vi "Measurement UI.vi"() -> ()   [LabVIEW 2021, in "ImageRendering.lvlib"]
uses:
  ImageRendering.lvlib
  <vilib>/vision/Image Controls.llb/IMAQ Image.ctl
  nivissvc.dll
  nivision.dll
panel:
  out "Time taken to receive image (seconds)":dbl
  out "Image Acq time":string
  out "Image Pixels (U32)":u32[](array[numeric])
  in  "Image Pixels (U64) 2":T1[][](array[typedef])
  in  "Image Converison Type":string(combo)="ImagePixelArray"
  out "Image Data Received":string
  out "value":u32[][](array[numeric])
  out "Image":T2(plugin-control)
  in  "Border Size":i32=3
  in  "Image Name":string="copy"
  in  "Image Type":u32(ring)=4 items=["Grayscale (U8)", "Grayscale (I16)", "Grayscale (SGL)", "Complex (CSG)", "RGB (U32)", "HSL (U32)", "RGB (U64)", "Grayscale (U16)"]
  out "File Size":dbl
  out "error out":errorcluster
  out "date/time string":string
  in  "Image Path":path
  out "Image Data":string
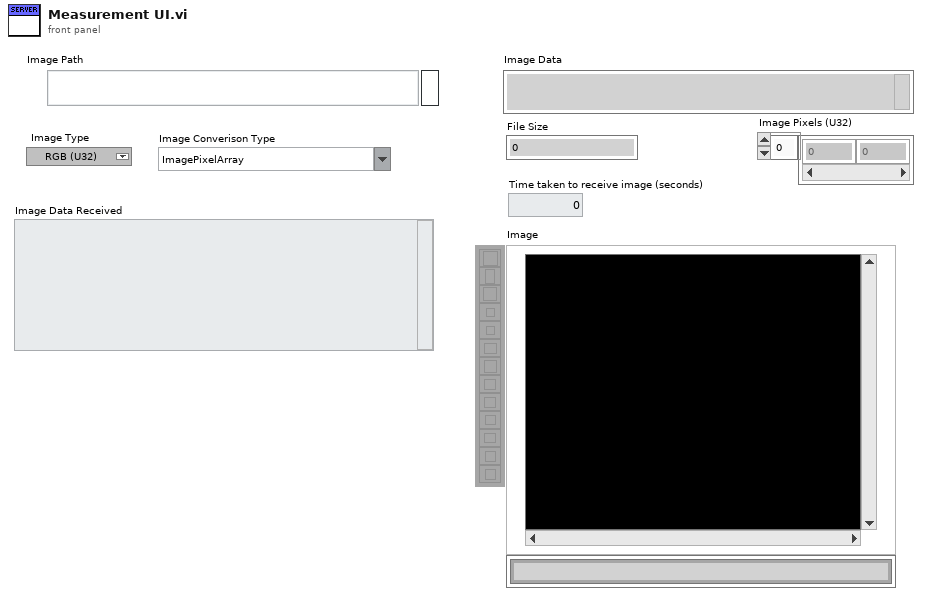
[diagram p1: front panel]
types:
  T1 = typedef "Color (U64)" = cluster{"Plane 3 (Blue)":u16, "Plane 2 (Green)":u16, "Plane 1 (Red)":u16, "Plane 4 (alpha)":u16}
  T2 = typedef "IMAQ Image.ctl" = refnum<image>
  T3 = enum16{"open", "replace", "create", "open or create", "replace or create", "replace or create with confirmation"}
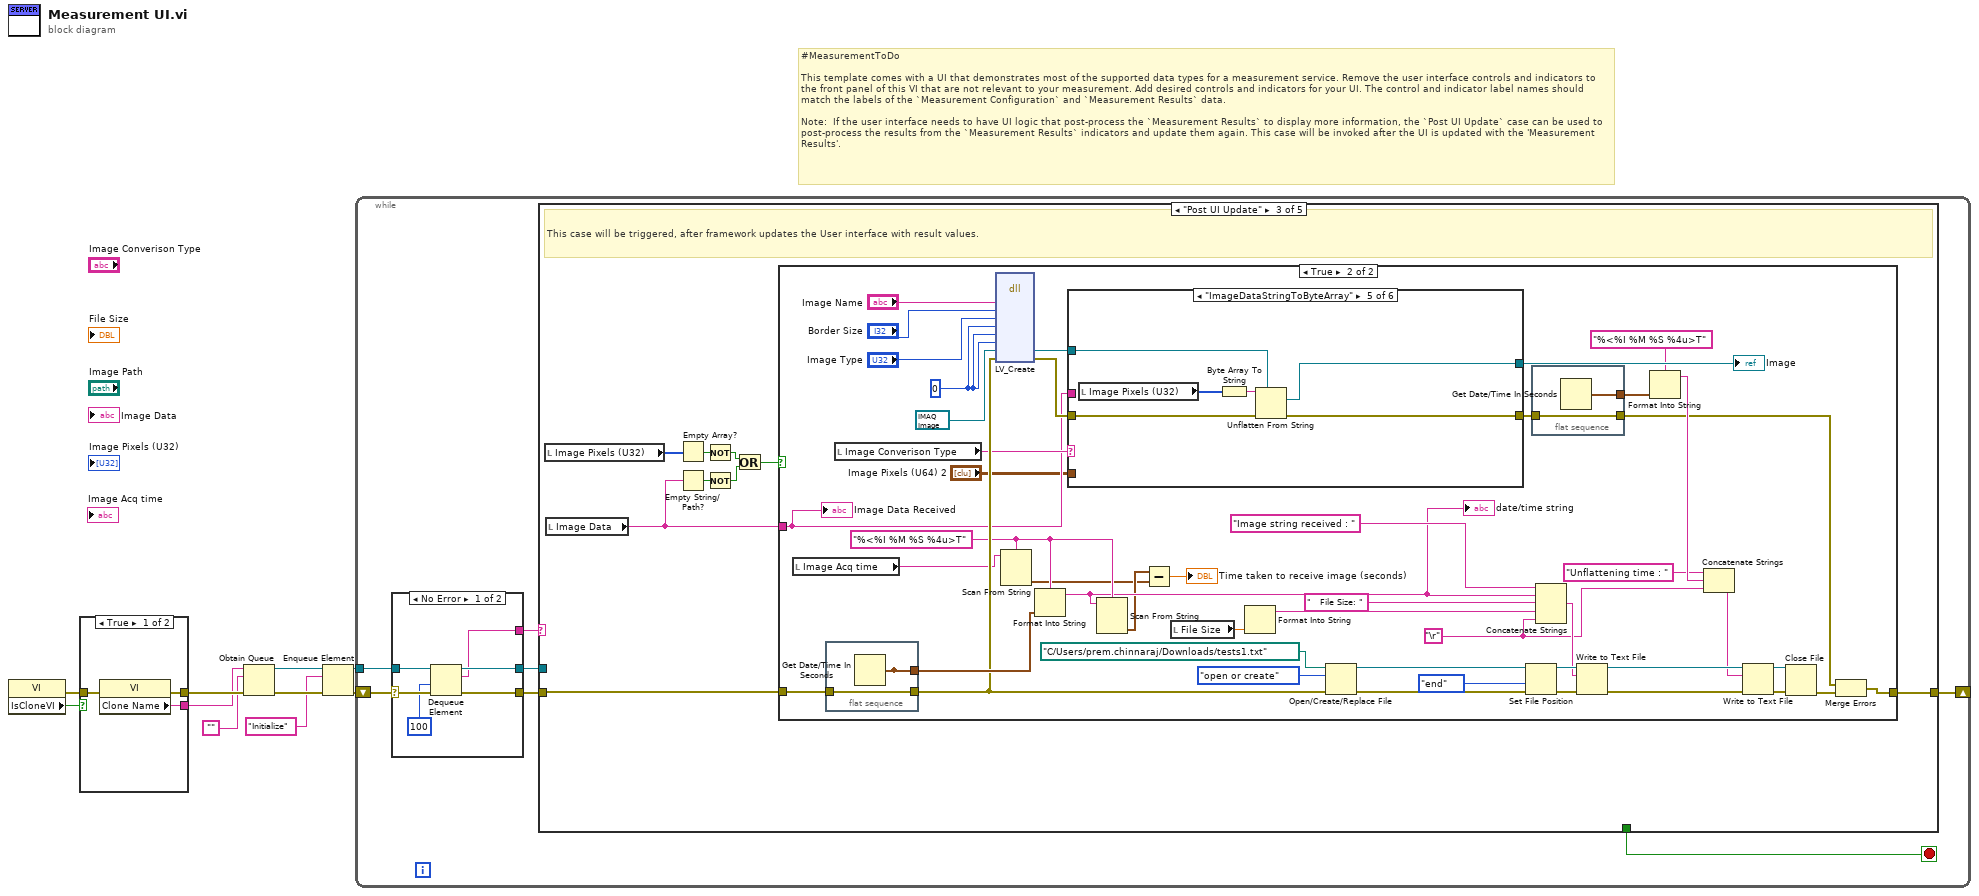
[diagram p0: block diagram]
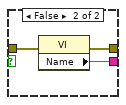
[diagram p2: hidden frame]
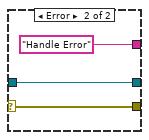
[diagram p3: hidden frame]
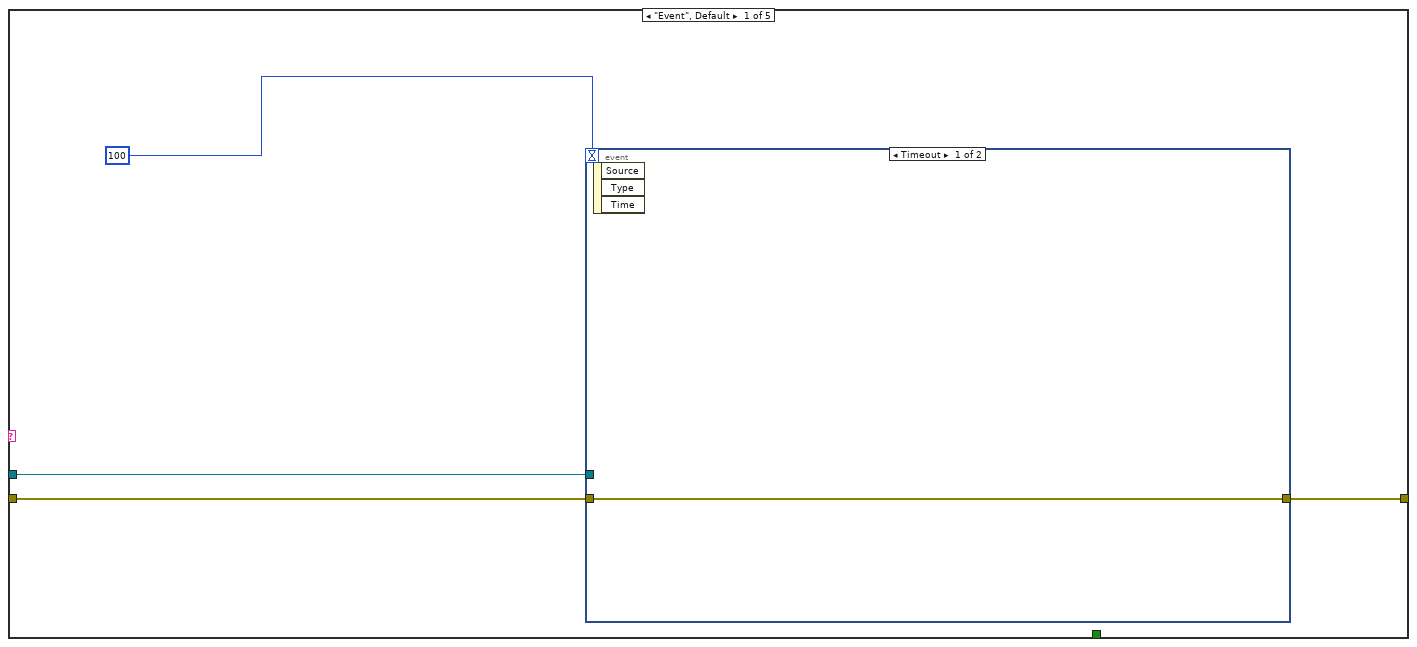
[diagram p4: hidden frame]
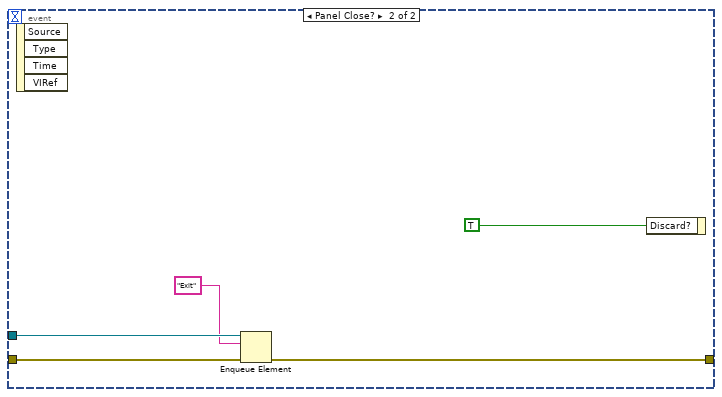
[diagram p5: hidden frame]
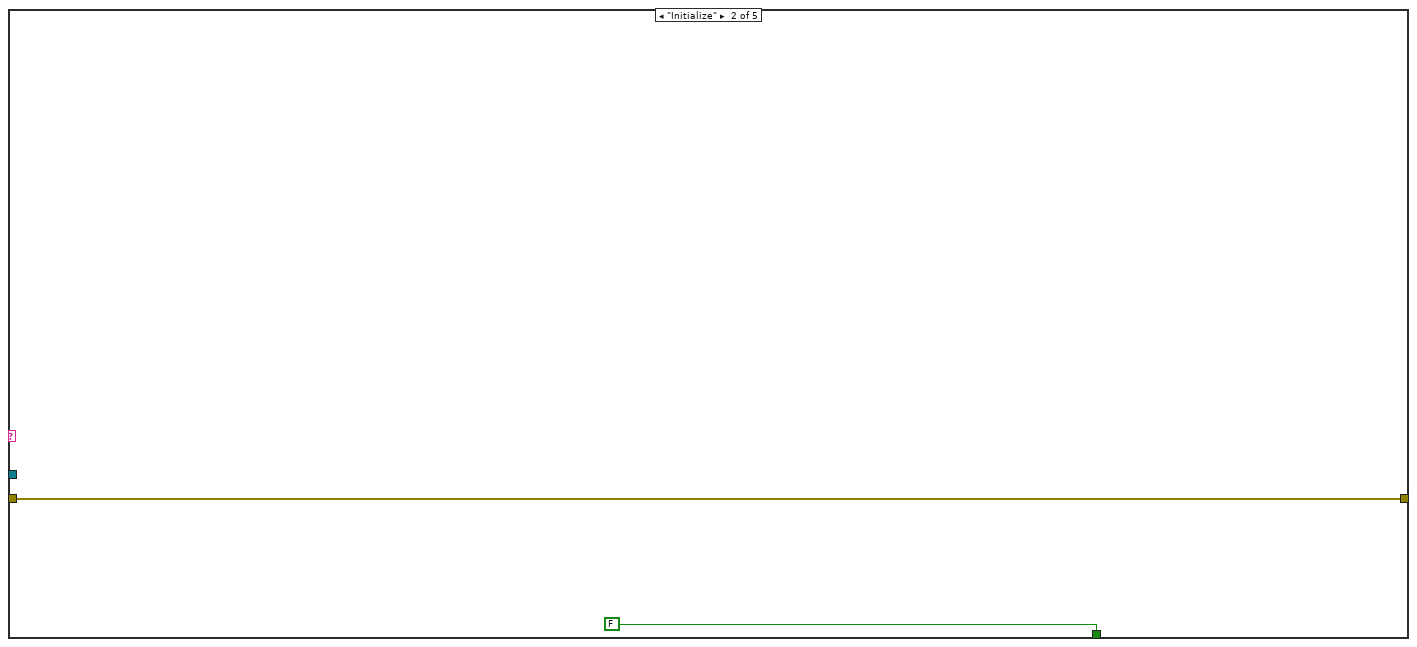
[diagram p6: hidden frame]
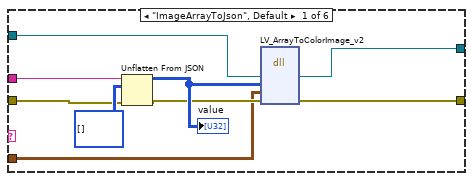
[diagram p8: hidden frame]
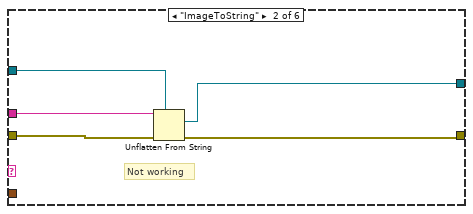
[diagram p9: hidden frame]
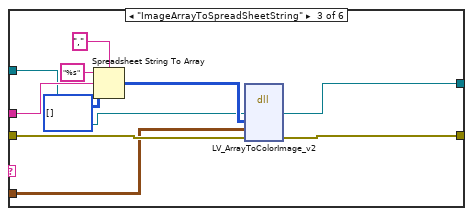
[diagram p10: hidden frame]
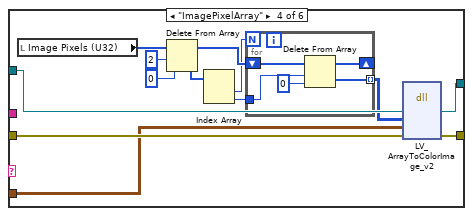
[diagram p11: hidden frame]
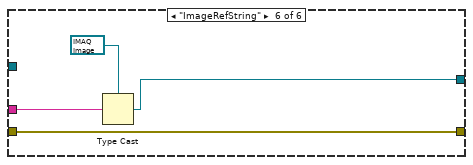
[diagram p12: hidden frame]
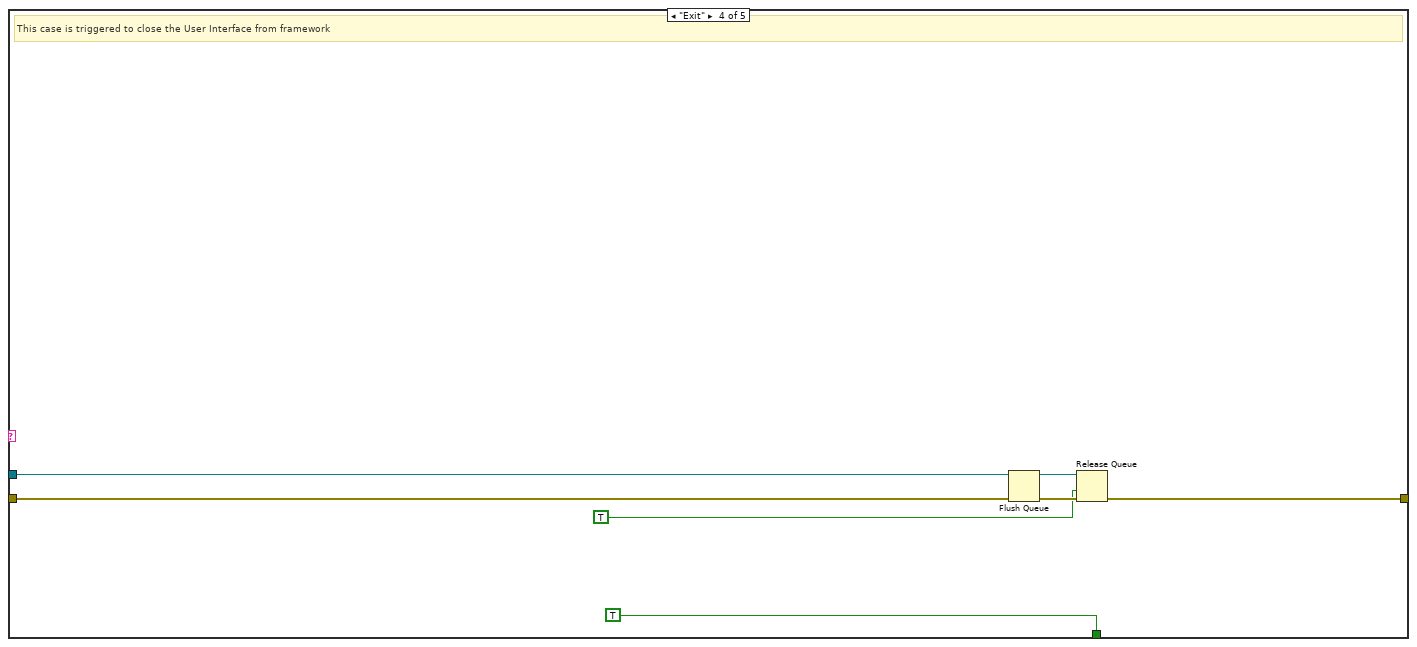
[diagram p13: hidden frame]
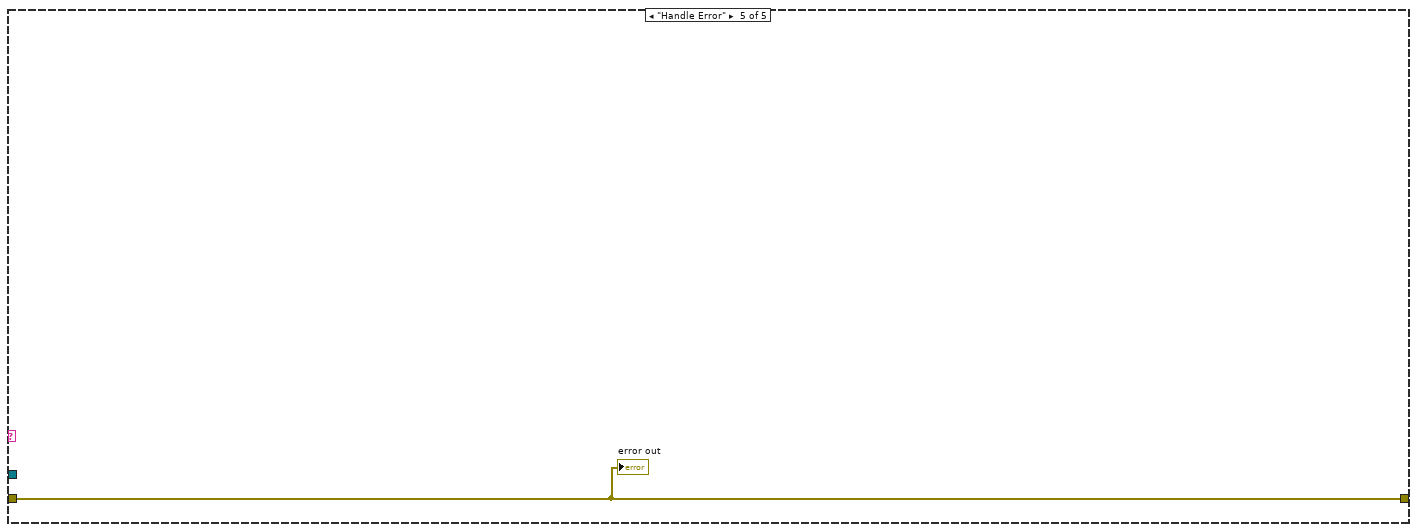
[diagram p14: hidden frame]
diagram:
  # "#MeasurementToDo  \n\nThis template comes with a UI that demonstrates most of the supported data types for a measurement service. Remove the user interface controls and indicators to the front panel of this VI that are not relevant to your measurement. Add desired controls and indicators for your UI. The control and indicator label names should match the labels of the `Measurement Configuration` and `Measurement Results` data.\n\nNote:  If the user interface needs to have UI logic that post-process the `Measurement Results` to display more information, the `Post UI Update` case can be used to post-process the results from the `Measurement Results` indicators and update them again. This case will be invoked after the UI is updated with the 'Measurement Results'."
  n1 = property class="VI"() -> (error out=w1:errorcluster, "IsCloneVI"=w2:bool)  [unwired: 2 in, 1 out]
  n2 = case shown="True" w2 {
    tunnel: [w13 w16] -> w10
    tunnel: [w12 w15] -> w9
    tunnel: w1 -> [w11 w14]
    frame True {
      n3 = property class="VI"(error in=w11) -> (error out=w13:errorcluster, "Clone Name"=w12:string)  [unwired: 1 in, 1 out]
    }
    frame False {
      n4 = property class="VI"(error in=w14) -> (error out=w16:errorcluster, "Name"=w15:string)  [unwired: 1 in, 1 out]
    }
  }
  n5 = Obtain Queue(name (unnamed)=w9, element data type="", error in (no error)=w10) -> (queue out=w6:refnum<queue>, error out=w8:errorcluster)  [unwired: 2 in, 1 out]
  n6 = Enqueue Element(queue=w6, element="Initialize", error in (no error)=w8) -> (queue out=w5:refnum<queue>, error out=w7:errorcluster)  [unwired: 1 in, 1 out]
  n7 = while {
    shift-right: [w19] -> _
    shift-left: w7 -> [w23]
    tunnel: w5 -> [w22]
    stop <- w18 stop-if-true
    n8 = case shown="No Error" w23 {
      selector: w23 -> [w29 w32]
      tunnel: [w28 w32] -> w17
      tunnel: w22 -> [w27 w31]
      tunnel: [w26 w31] -> w21
      tunnel: [w25 "Handle Error"] -> w20
      frame No Error {
        n9 = Dequeue Element(queue=w27, timeout in ms (-1)=100, error in (no error)=w29) -> (queue out=w26:refnum<queue>, element=w25:string, error out=w28:errorcluster)  [unwired: 1 out]
      }
      frame Error {
      }
    }
    n10 = case shown="\"Post UI Update\"" w20 {
      tunnel: w17 -> [w35 w44 w52 w163 w164]
      tunnel: w21 -> [w33 _ _ w161 _]
      tunnel: [w36 w44 w53 w158 w164] -> w19
      tunnel: [_ FALSE _ TRUE _] -> w18
      frame "Event", Default {
        n11 = event shown="[0] Timeout" {
          selector: _ -> [_ _]
          dyn-events: _ -> [_ _]
          timeout: 100 -> [_ _]
          tunnel: [w37 w40] -> w36
          tunnel: w35 -> [w37 w41]
          tunnel: w33 -> [_ w39]
          event Timeout {
            n12 = event-data() -> ()  [unwired: 1 in, 3 out]
          }
          event Panel Close? {
            n13 = event-data() -> ()  [unwired: 1 in, 4 out]
            n14 = Enqueue Element(queue=w39, element="Exit", error in (no error)=w41) -> (error out=w40:errorcluster)  [unwired: 1 in, 2 out]
            n15 = event-data("Discard?"=TRUE) -> ()  [unwired: 1 in, 1 out]
          }
        }
      }
      frame "Initialize" {
      }
      frame "Post UI Update" {
        # "This case will be triggered, after framework updates the User interface with result values."
        n16 = local read "Image Pixels (U32)"() -> (w50:u32[])
        n17 = local read "Image Data"() -> (w48:string)
        n18 = Empty Array?(array=w50) -> (empty?=w51:bool)
        n19 = Empty String/Path?(string/path=w48) -> (empty?=w47:bool)
        n20 = Not(x=w51) -> (.not. x?=w49:bool)
        n21 = Not(x=w47) -> (.not. x?=w46:bool)
        n22 = Or(x=w49, y=w46) -> (x .or. y?=w45:bool)
        n23 = case shown="True" w45 {
          tunnel: [w54 w62] -> w53
          tunnel: w52 -> [w54 w69]
          tunnel: w48 -> [_ w64]
          frame False {
          }
          frame True {
            w59 = "%<%I %M %S %4u>T" ("format string")
            w84 = 0
            w72 = "\r"
            n24 = local read "Image Acq time"() -> (w60:string)
            n25 = flat-sequence {
              tunnel: w69 -> [w154]
              tunnel: [w154] -> w66
              tunnel: [w153] -> _
              tunnel: [w153] -> w68
              frame #0 {
                n26 = Get Date/Time In Seconds() -> (seconds since 1Jan1904=w153:timestamp)
              }
            }
            n27 = local read "Image Converison Type"() -> (w65:string)
            n28 = dll-call lib="nivissvc.*" fn="LV_Create"("name"="Image Name", "border"="Border Size", "imageType"="Image Type", "width"=w84, "height"=w84, "lock space"=w84, "image"=T2 refnum ("New Image"), "error out 2"=w66) -> ("image"=w82:T2, "error out 2"=w67:errorcluster)  [unwired: 9 in, 3 out]
            n29 = Scan From String(format string=w59, input string=w60) -> (output 1=w56:timestamp)  [unwired: 3 in, 3 out]
            n30 = Format Into String(format string=w59, w68) -> (resulting string=w58:string)  [unwired: 2 in, 1 out]
            "date/time string" <- w58
            n31 = case shown="\"ImageDataStringToByteArray\"" w65 {
              tunnel: w64 -> [w109 w112 w124 _ _ w151]
              tunnel: w82 -> [w106 w111 w117 w135 w144 _]
              tunnel: [w105 w110 w116 w134 w143 w150] -> w81
              tunnel: [w104 w113 w120 w136 w146 w152] -> w76
              tunnel: w67 -> [w103 w114 w121 w137 w148 w152]
              tunnel: "Image Pixels (U64) 2" -> [w101 _ w115 w133 _ _]
              frame "ImageArrayToJson", Default {
                n32 = Unflatten From JSON(JSON string=w109, type and defaults=u32[][] [] ("Image Pixels (U32)"), error in (no error)=w103) -> (value=w107:u32[][], error out=w102:errorcluster)  [unwired: 4 in]
                "value" <- w107
                n33 = dll-call lib="nivision.*" fn="LV_ArrayToColorImage_v2"("image"=w106, "array32"=w107, "array64"=w101, "error"=w102) -> ("image"=w105:T2, "error"=w104:errorcluster)  [unwired: 5 in, 3 out]
              }
              frame "ImageToString" {
                # "Not working"
                n34 = Unflatten From String(type=w111, binary string=w112, error in (no error)=w114) -> (value=w110:T2, error out=w113:errorcluster)  [unwired: 2 in, 1 out]
              }
              frame "ImageArrayToSpreadSheetString" {
                n35 = Spreadsheet String To Array(delimiter (Tab)=",", format string="%s", spreadsheet string=w124, array type (2D Dbl)=u32[][] [] ("Image Pixels (U32)")) -> (array=w119:u32[][])
                n36 = dll-call lib="nivision.*" fn="LV_ArrayToColorImage_v2"("image"=w117, "array32"=w119, "array64"=w115, "error"=w121) -> ("image"=w116:T2, "error"=w120:errorcluster)  [unwired: 5 in, 3 out]
              }
              frame "ImagePixelArray" {
                n37 = local read "Image Pixels (U32)"() -> (w132:u32[])
                n38 = Delete From Array(array=w132, length=2, index=0) -> (deleted portion=w128:u32[], array with subset deleted=w129:u32[])
                n39 = Index Array(array=w128) -> (element #1=w127:u32, element #2=w126:u32)  [unwired: 2 in]
                n40 = for {
                  N: w127 -> [_]
                  tunnel: w126 -> [w142]
                  shift-right: [w139] -> _
                  shift-left: w129 -> [w140]
                  tunnel: [w138] -> w125 mode=indexing
                  n41 = Delete From Array(array=w140, length=w142, index=0) -> (deleted portion=w138:u32[], array with subset deleted=w139:u32[])
                }
                n42 = dll-call lib="nivision.*" fn="LV_ArrayToColorImage_v2"("image"=w135, "array32"=w125, "array64"=w133, "error"=w137) -> ("image"=w134:T2, "error"=w136:errorcluster)  [unwired: 5 in, 3 out]
              }
              frame "ImageDataStringToByteArray" {
                n43 = local read "Image Pixels (U32)"() -> (w147:u32[])
                n44 = Byte Array To String(unsigned byte array=w147) -> (string=w145:string)
                n45 = Unflatten From String(type=w144, binary string=w145, error in (no error)=w148) -> (value=w143:T2, error out=w146:errorcluster)  [unwired: 2 in, 1 out]
              }
              frame "ImageRefString" {
                n46 = Type Cast(type=T2 refnum ("New Image"), x=w151) -> (*(type *) &x=w150:T2)
              }
            }
            "Image" <- w81
            n47 = Scan From String(format string=w59, input string=w58) -> (output 1=w57:timestamp)  [unwired: 3 in, 3 out]
            n48 = Subtract(x=w57, y=w56) -> (x-y=→"Time taken to receive image (seconds)":dbl)
            n49 = local read "File Size"() -> (w89:dbl)
            n50 = Format Into String(w89) -> (resulting string=w88:string)  [unwired: 3 in, 1 out]
            n51 = Open/Create/Replace File(file path (use dialog)=path "C:/Users/prem.chinnaraj/Downloads/tests1.txt" ("file (use dialog)"), error in=w66, operation (0:open)=T3."open or create") -> (refnum out=w93:refnum<file>, error out=w100:errorcluster)  [unwired: 3 in, 1 out]
            n52 = Set File Position(refnum=w93, from (0:start)=enum16{"start", "end", "current"}."end", error in=w100) -> (refnum out=w92:refnum<file>, error out=w94:errorcluster)  [unwired: 1 in]
            n53 = flat-sequence {
              tunnel: w76 -> [w156]
              tunnel: [w156] -> w61
              tunnel: [w155] -> w74
              frame #0 {
                n54 = Get Date/Time In Seconds() -> (seconds since 1Jan1904=w155:timestamp)
              }
            }
            n55 = Concatenate Strings("Image string received : " ("string"), w58, "   File Size: " ("string"), w88, w72) -> (w77:string)
            n56 = Write to Text File(file (use dialog)=w92, text=w77, error in=w94) -> (refnum out=w79:refnum<file>, error out=w99:errorcluster)  [unwired: 1 in, 1 out]
            n57 = Format Into String(format string="%<%I %M %S %4u>T", w74) -> (resulting string=w73:string)  [unwired: 2 in, 1 out]
            n58 = Concatenate Strings("Unflattening time : " ("string"), w73, w72) -> (w70:string)
            n59 = Write to Text File(file (use dialog)=w79, text=w70, error in=w99) -> (refnum out=w78:refnum<file>, error out=w80:errorcluster)  [unwired: 1 in, 1 out]
            n60 = Close File(refnum=w78, error in=w80) -> (error out=w95:errorcluster)  [unwired: 1 out]
            n61 = Merge Errors(w61, w95) -> (w62:errorcluster)
            "Image Data Received" <- w64
          }
        }
      }
      frame "Exit" {
        # "This case is triggered to close the User Interface from framework"
        n62 = Flush Queue(queue=w161, error in (no error)=w163) -> (queue out=w160:refnum<queue>, error out=w159:errorcluster)  [unwired: 1 out]
        n63 = Release Queue(queue=w160, force destroy? (F)=TRUE, error in (no error)=w159) -> (error out=w158:errorcluster)  [unwired: 2 out]
      }
      frame "Handle Error" {
        "error out" <- w164
      }
    }
  }
